vi "09_combined_example.vi"() -> ()   [LabVIEW 2018, in "LV-0mq-Julia_roundtrip-lib.lvlib" / "LV2Julia_examples.lvlib"]
uses:
  LV2Julia_examples.lvlib
  LV2Julia_core/VIs/Server or client state.ctl
  LV2Julia_core/VIs/detailed error info.ctl
  LV2Julia_core/VIs/StackFrame.ctl
  simple examples functions.ctl
  LV2Julia_core/VIs/Commands.ctl
  edf81fa3-46bf-427f-9605-85b461656974.vi
  29886417-d43f-41fb-9c0c-469db3f8c96d.vi
  3fe35f36-217a-40a5-a789-8326c52a1f5c.vi
  35a44a82-786b-41ea-be73-9a4468e4df9d.vi
  edf81fa3-46bf-427f-9605-85b461656974.vi/d78438c1-e9c2-4049-8a01-ea359766d27e.vi
  29886417-d43f-41fb-9c0c-469db3f8c96d.vi/726a0e03-44e9-4b5b-8c33-3fdb3adf96f2.vi
  3fe35f36-217a-40a5-a789-8326c52a1f5c.vi/be66880e-2f9f-43fa-8a25-3020ddce25df.vi
  35a44a82-786b-41ea-be73-9a4468e4df9d.vi/e765cad0-9840-4168-a112-da73896eb643.vi
  35a44a82-786b-41ea-be73-9a4468e4df9d.vi/f3238023-a8b3-435f-be8b-4be774610aa1.vi
  edf81fa3-46bf-427f-9605-85b461656974.vi/d78438c1-e9c2-4049-8a01-ea359766d27e.vi/edf13171-bb8c-4b0e-8a13-cfaee6010a46.vi
  29886417-d43f-41fb-9c0c-469db3f8c96d.vi/726a0e03-44e9-4b5b-8c33-3fdb3adf96f2.vi/e7bf7d0e-5fa3-492d-91d8-494ec4c78bd1.vi
  29886417-d43f-41fb-9c0c-469db3f8c96d.vi/726a0e03-44e9-4b5b-8c33-3fdb3adf96f2.vi/bcfacdb4-d734-4844-97c1-59f988d0ab4b.vi
  29886417-d43f-41fb-9c0c-469db3f8c96d.vi/726a0e03-44e9-4b5b-8c33-3fdb3adf96f2.vi/27f03db2-f0c9-44fc-95a3-84f8622bf8b3.vi
  3fe35f36-217a-40a5-a789-8326c52a1f5c.vi/be66880e-2f9f-43fa-8a25-3020ddce25df.vi/b22e8afe-8408-4b96-ba33-df0573f8bda9.vi
  3fe35f36-217a-40a5-a789-8326c52a1f5c.vi/be66880e-2f9f-43fa-8a25-3020ddce25df.vi/973810d6-8273-42e9-becd-a912c4fb1f62.vi
  3fe35f36-217a-40a5-a789-8326c52a1f5c.vi/be66880e-2f9f-43fa-8a25-3020ddce25df.vi/742d8af4-4bb6-4e08-85d7-281a839dc2ce.vi
  35a44a82-786b-41ea-be73-9a4468e4df9d.vi/e765cad0-9840-4168-a112-da73896eb643.vi/dc34fd2d-f794-448f-aba6-043ae9d4d40f.vi
  35a44a82-786b-41ea-be73-9a4468e4df9d.vi/e765cad0-9840-4168-a112-da73896eb643.vi/fa03b5a1-01ca-4e07-872a-a6bd434a2e33.vi
  edf81fa3-46bf-427f-9605-85b461656974.vi/d78438c1-e9c2-4049-8a01-ea359766d27e.vi/edf13171-bb8c-4b0e-8a13-cfaee6010a46.vi/3952a552-d88b-4b70-b2de-8936c03ae8d7.vi
  35a44a82-786b-41ea-be73-9a4468e4df9d.vi/e765cad0-9840-4168-a112-da73896eb643.vi/dc34fd2d-f794-448f-aba6-043ae9d4d40f.vi/6b1990a7-d1b9-4824-acae-e43fafbf4c5e.vi
  LV2Julia_core/VIs/jl-scripts path.vi
  LV2Julia_core/VIs/check ID validity.vi
  LV2Julia_core/VIs/bindata_descr to JSON.vi
  LV2Julia_core/VIs/check cluster field names.vi
  LV2Julia_core/VIs/concat JSON.vi
  LV2Julia_core/VIs/build request.vi
  LV2Julia_core/VIs/Parse server response.vi
  LV2Julia_core/VIs/log jl exceptions.vi
  <vilib>/Utility/error.llb/Error Cluster From Error Code.vi
  LV2Julia_core/LV2Julia_core.lvlib
  <vilib>/measure/NI_MABase.lvlib
panel:
  out "ZMQ timeout":bool
  out "Julia script file path":path
  out "temporary script path":path
  out "Jl Server state":T1
  in  "execution control pages":enum32{"Start", "go - test"}(tab)
  in  "go":bool caption="go (Julia Server started externally)"
  in  "Start with Julia":bool caption="Start Julia Server and go"
  in  "ZMQ endpoint":string="tcp://127.0.0.1:5555"
  in  "p":dbl=1.0
  in  "fn":T2 caption="select function at Server" items=["arr_amplitude", "arr_length", "arr_mean", "arr_median", "arr_rms", "vec_amplify", "vec_attenuate", "vec_power"]
  in  "trim @ begin":dbl
  in  "trim @ end":dbl
  in  "Group":T3(tab)
  out "Server response":dbl
  out "data received plot":dbl[](graph)
  out "data received":dbl[](array[numeric]) format="%.3f"
  out "RMS":dbl
  out "detailed error info":T4
  out "current error":errorcluster
  out "final error":errorcluster
  out "short err code":u8
  in  "tones":T6(array[cluster])=[{"frequency"=10.0, "amplitude"=1.0, "phase"=0.0}, {"frequency"=20.0, "amplitude"=0.1, "phase"=0.0}] {"phase" format="%.2p"; "amplitude" format="%0.2p"; "frequency" format="%0.2p"}
  in  "noise (rms)":dbl=0.1 format="%.2p"
  in  "offset":dbl format="%.2p"
  in  "sampling info":cluster{"Fs":dbl, "#s":dbl}={"Fs"=1000.0, "#s"=1000.0} {"Fs" format="%.2p"}
  in  "next":bool
  out "data sent to server":dbl[](graph)
  out "data sent":dbl[](array[numeric]) format="%.3f"
  out "function name":string
  in  "stop this VI only":bool
  in  "stop both this VI and Julia Server":bool
  # "tcp://127.0.0.1:5555 \nfor local Julia Server\n\nFor a Julia Server running on a separate computer,  you probably must use an IPv4 address in numeric form (not a DNS name) - see https://stackoverflow.com/questions/6024003/why-doesnt-zeromq-work-on-localhost.\n\nThis control only used if Julia Server is not being started by this VI."
  # "generate sample array"
  # "function and parameter"
  # "enter a negative or a large positive value to cause an exception"
  # "data returned by server"
  # "data sent to server"
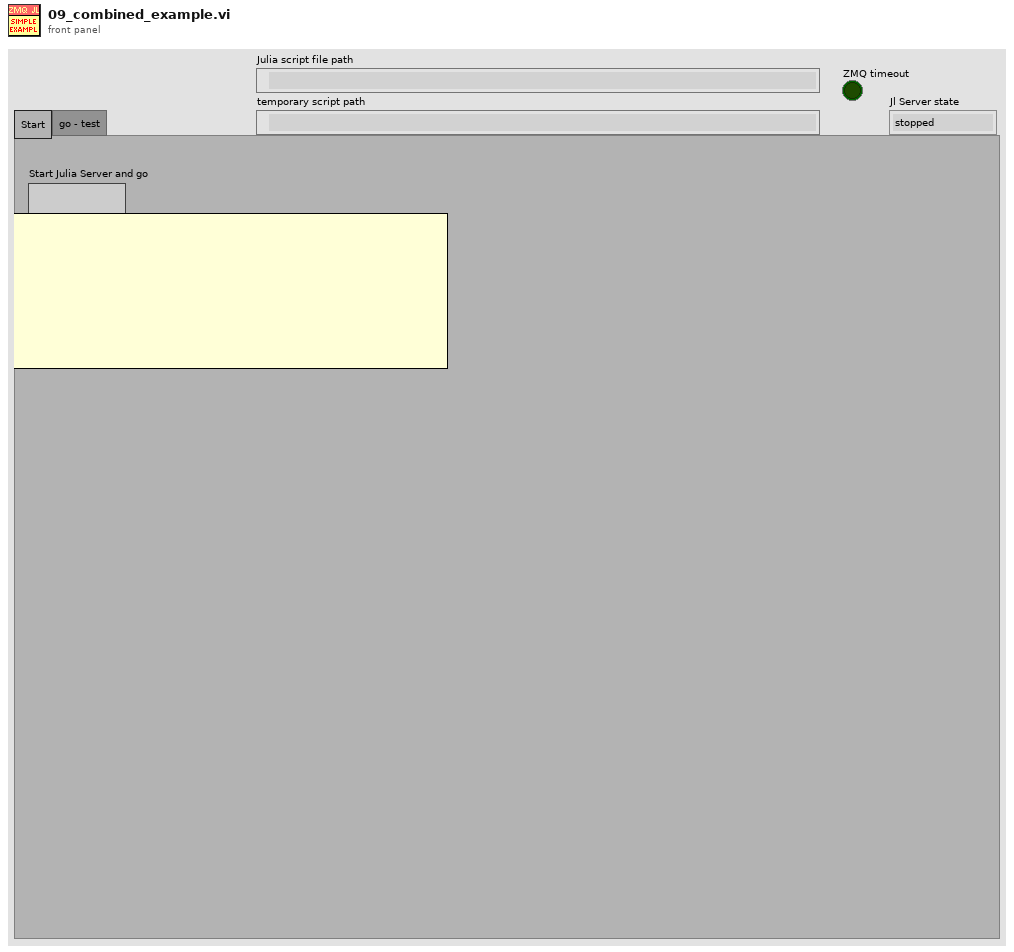
[diagram p1: front panel]
types:
  T1 = typedef "LV-0mq-Julia_roundtrip-lib.lvlib/LV2Julia_core.lvlib/Server or client state.ctl" = enum16{"stopped", "running", "unknown"}
  T2 = typedef "LV-0mq-Julia_roundtrip-lib.lvlib/LV2Julia_examples.lvlib/simple examples functions.ctl" = u16
  T3 = enum32{"fns returning scalar", "fns returning vector", "error"}
  T4 = typedef "LV-0mq-Julia_roundtrip-lib.lvlib/LV2Julia_core.lvlib/detailed error info.ctl" = cluster{"exception_or_info":string, "trace":T5[]}
  T5 = typedef "LV-0mq-Julia_roundtrip-lib.lvlib/LV2Julia_core.lvlib/StackFrame.ctl" = cluster{"frame_summary":string, "func":string, "linfo":string, "file":string, "line":i32, "pointer":u64, "from_c":bool, "inlined":bool}
  T6 = cluster{"frequency":dbl, "amplitude":dbl, "phase":dbl}[]
  T7 = typedef "LV-0mq-Julia_roundtrip-lib.lvlib/LV2Julia_core.lvlib/Commands.ctl" = enum16{"Start Jl-server & Init LV-client", "Send request & Get response ", "Stop Jl-server & Cleanup LV-client", "Cleanup LV-client", "Start Jl-server", "Stop Jl-server", "Init LV-Client", "Cleanup LV-Client", "(not allowed)", "Set LV Client state", "Set Jl Server state", "set ZMQ timeout", "read ZMQ timeout", "read-out state"}
  T8 = enum8{"Enabled", "Disabled", "Disabled and Grayed Out"}
  T9 = typedef "LV-0mq-Julia_roundtrip-lib.lvlib/LV2Julia_core.lvlib/Bindata&description.ctl" = cluster{"bindata_descr":T10[], "bindata":u8[]}
  T10 = typedef "LV-0mq-Julia_roundtrip-lib.lvlib/LV2Julia_core.lvlib/Bindata description.ctl" = cluster{"nofbytes":i32, "numtype":string, "start":i32, "arrdims":i32[], "kwarg_name":string, "category":string}
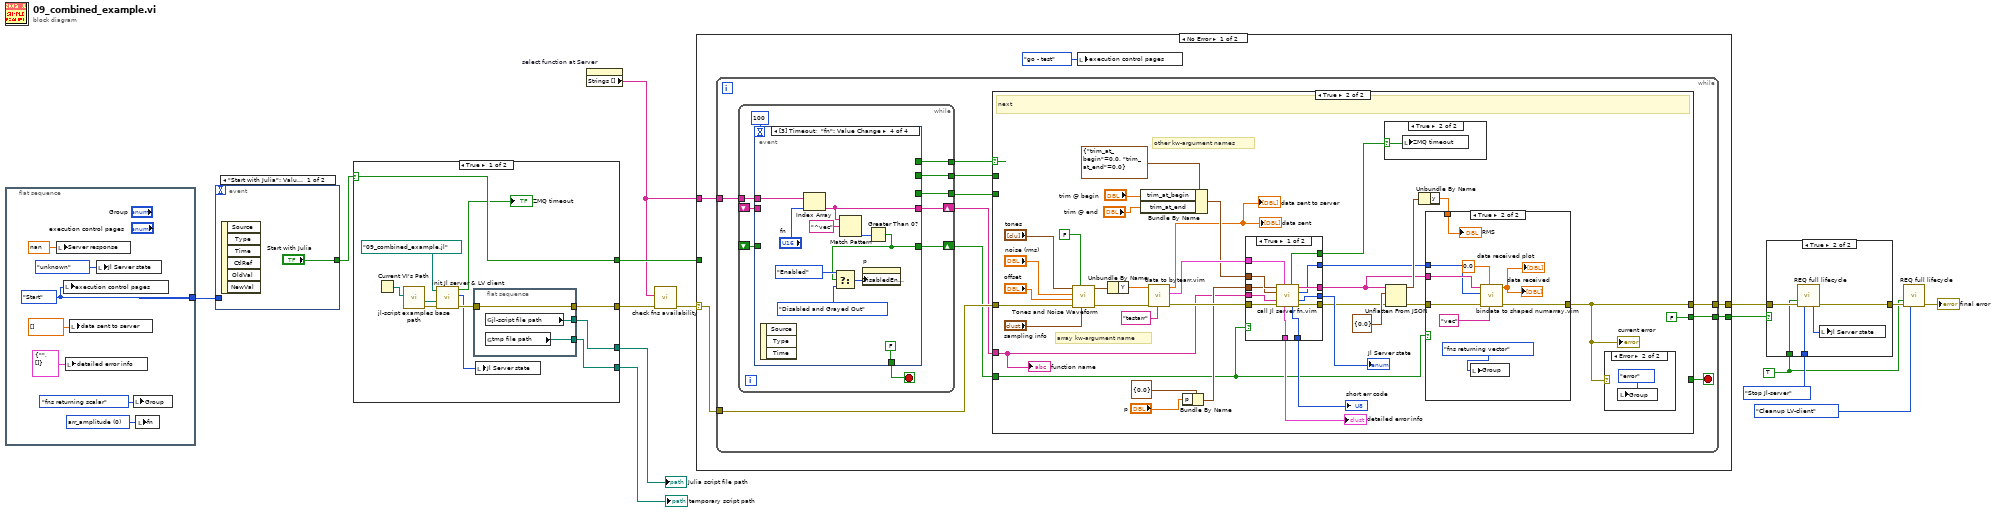
[diagram p0: block diagram]
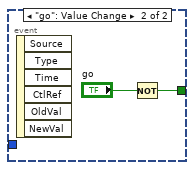
[diagram p2: hidden frame]
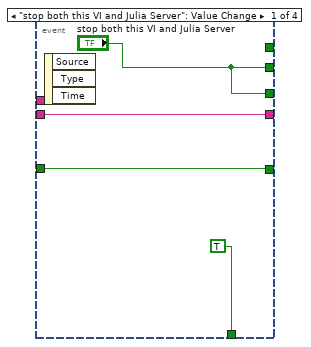
[diagram p3: hidden frame]
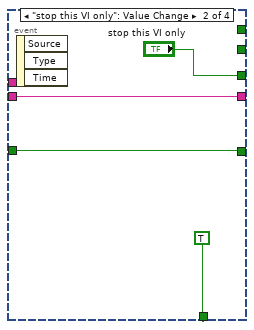
[diagram p4: hidden frame]
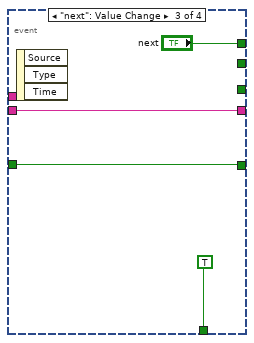
[diagram p5: hidden frame]
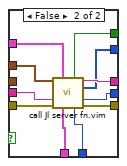
[diagram p7: hidden frame]
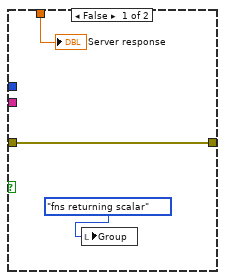
[diagram p9: hidden frame]
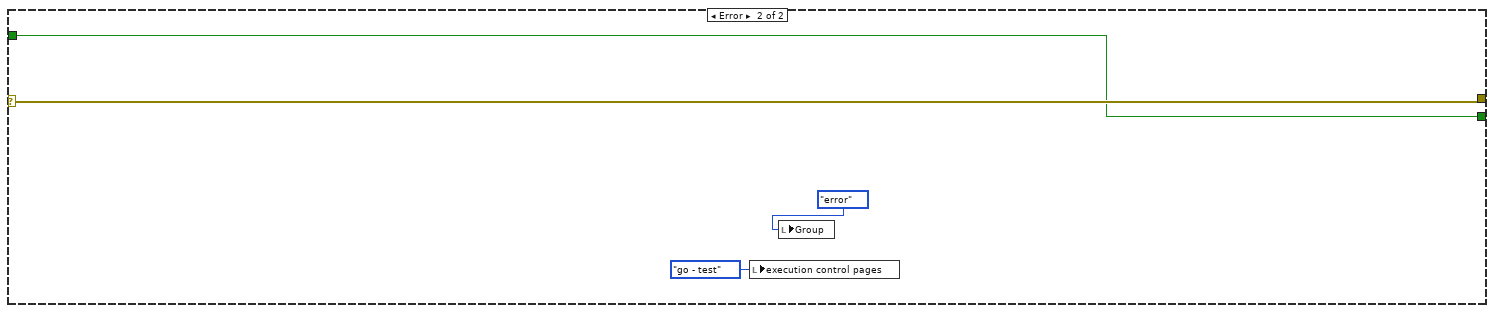
[diagram p11: hidden frame]
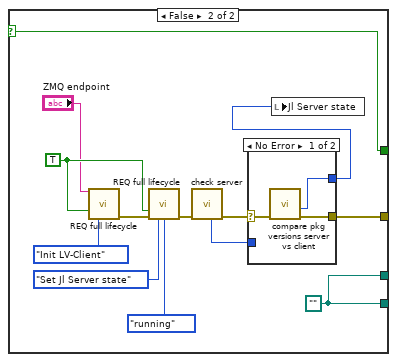
[diagram p12: hidden frame]
diagram:
  w10 = TRUE ("Force command")
  n1 = flat-sequence {
    tunnel: [w22] -> w6
    frame #0 {
      w16 = T2 0 items=["arr_amplitude", "arr_length", "arr_mean", "arr_median", "arr_rms", "vec_amplify", "vec_attenuate", "vec_power"] ("fn")
      w22 = enum32{"Start", "go - test", "finish"}."Start" ("execution control pages")
      n2 = local write "Server response"(nan ("Server response")) -> ()
      n3 = local write "execution control pages"(w22) -> ()
      n4 = local write "detailed error info"(T4 {"exception_or_info"="", "trace"=[]} ("detailed error info")) -> ()
      n5 = local write "data sent to server"(dbl[] []) -> ()
      n6 = local write "Jl Server state"(Server_or_client_state."unknown" ("Jl Server state out")) -> ()
      n7 = local write "Group"(T3."fns returning scalar" ("Group")) -> ()
      n8 = local write "fn"(w16) -> ()
    }
  }
  n9 = event shown="[0] \"Start with Julia\": Value Change" {
    selector: _ -> [_ _]
    dyn-events: _ -> [_ _]
    timeout: _ -> [_ _]
    tunnel: ["Start with Julia" w24] -> w8
    tunnel: w6 -> [_ _]
    event "Start with Julia": Value Change {
      n10 = event-data() -> ()  [unwired: 1 in, 6 out]
    }
    event "go": Value Change {
      n11 = event-data() -> ()  [unwired: 1 in, 6 out]
      n12 = Not(x="go") -> (.not. x?=w24:bool)
    }
  }
  n13 = case shown="True" w8 {
    selector: w8 -> [w36 w48]
    tunnel: [w35 w42] -> w5
    tunnel: [w36 w48] -> w7
    tunnel: [w34 w45] -> w1
    tunnel: [w33 w45] -> w2
    frame True {
      n14 = Current VI's Path() -> (path=w28:path)
      n15 = call "jl-script examples base path.vi"("calling example VI path"=w28) -> ("error out"=w27:errorcluster, "jl-script-examples base path"=w26:path)  [unwired: 9 in]
      n16 = call "init Jl server & LV client.vi"("error in (no error)"=w27, "Base path (not a path)"=w26, "Julia user functions script"=path "09_combined_example.jl") -> ("error out"=w30:errorcluster, "Jl Server state out"=w29:T1, "timeout?"=→"ZMQ timeout":bool)  [unwired: 6 in]
      n17 = flat-sequence {
        tunnel: [w39] -> w35
        tunnel: w30 -> [w39]
        tunnel: [w38] -> w34
        tunnel: [w37] -> w33
        frame #0 {
          n18 = global read "jl-scripts path.vi" "jl-script file path"() -> (w38:path)
          n19 = global read "jl-scripts path.vi" "tmp file path"() -> (w37:path)
        }
      }
      n20 = local write "Jl Server state"(w29) -> ()
    }
    frame False {
      w45 = path ""
      w50 = TRUE ("Force command")
      n21 = call "REQ full lifecycle.vi"("ZMQ endpoint"="ZMQ endpoint", "Force command"=w50, "command"=Commands."Init LV-Client") -> ("error out"=w47:errorcluster)  [unwired: 6 in, 6 out]
      n22 = call "REQ full lifecycle.vi"("Force command"=w50, "error in"=w47, "command"=Commands."Set Jl Server state", "Jl Server state in"=Server_or_client_state."running") -> ("error out"=w46:errorcluster)  [unwired: 5 in, 6 out]
      n23 = call "check server.vi"("error in"=w46) -> ("error out"=w43:errorcluster, "Jl Server state out"=w41:T1)  [unwired: 6 in, 3 out]
      n24 = case shown="No Error" w43 {
        selector: w43 -> [w55 w57]
        tunnel: [w54 w57] -> w42
        tunnel: [w53 w56] -> w40
        tunnel: w41 -> [_ w56]
        frame No Error {
          n25 = call "compare pkg versions server vs client.vi"("error in (no error)"=w55) -> ("error out"=w54:errorcluster, "Jl Server state out"=w53:T1)  [unwired: 4 in, 5 out]
        }
        frame Error {
        }
      }
      n26 = local write "Jl Server state"(w40) -> ()
    }
  }
  "temporary script path" <- w2
  "Julia script file path" <- w1
  n27 = property on="select function at Server" class="Ring (strict)"() -> ("Strings []"=w3:string[])  [unwired: 2 in, 2 out]
  n28 = call "check fns availability.vi"("error in (no error)"=w5, "fns list is"=w3) -> ("error out"=w4:errorcluster)  [unwired: 3 in, 6 out]
  n29 = case shown="No Error" w4 {
    selector: w4 -> [w61 w183]
    tunnel: [w62 w183] -> w15
    tunnel: [w60 w182] -> w9
    tunnel: w3 -> [w59 _]
    tunnel: w7 -> [_ w182]
    frame No Error {
      n30 = while {
        tunnel: w61 -> [w71]
        tunnel: [w72] -> w62
        tunnel: [w68] -> w60
        tunnel: w59 -> [w66]
        stop <- w69 stop-if-true
        n31 = while {
          tunnel: [w82] -> w70
          tunnel: [w81] -> w67
          tunnel: w66 -> [w78]
          shift-right: [w77] -> w65
          shift-left: _ -> [w74]
          shift-right: [w76] -> w64
          shift-left: _ -> [w75]
          tunnel: [w73] -> w63
          stop <- w80 stop-if-true
          n32 = event shown="[3] Timeout;  \"fn\": Value Change" {
            selector: _ -> [_ _ _ _]
            dyn-events: _ -> [_ _ _ _]
            timeout: 100 -> [_ _ _ _]
            tunnel: ["stop both this VI and Julia Server" _ _ _] -> w81
            tunnel: [_ _ "next" _] -> w82
            tunnel: [TRUE TRUE TRUE FALSE] -> w80
            tunnel: w78 -> [_ _ _ w98]
            tunnel: [w84 w88 w92 w97] -> w77
            tunnel: [w85 w89 w91 w96] -> w76
            tunnel: w75 -> [w85 w89 w91 _]
            tunnel: w74 -> [w84 w88 w92 _]
            tunnel: ["stop both this VI and Julia Server" "stop this VI only" _ _] -> w73
            event "stop both this VI and Julia Server": Value Change {
              n33 = event-data() -> ()  [unwired: 1 in, 3 out]
            }
            event "stop this VI only": Value Change {
              n34 = event-data() -> ()  [unwired: 1 in, 3 out]
            }
            event "next": Value Change {
              n35 = event-data() -> ()  [unwired: 1 in, 3 out]
            }
            event Timeout; Value Change {
              n36 = event-data() -> ()  [unwired: 1 in, 3 out]
              n37 = Index Array(array=w98, index="fn") -> (element=w96:string)
              n38 = Match Pattern(string=w96, regular expression="^vec") -> (offset past match=w102:i32)  [unwired: 1 in, 3 out]
              n39 = Greater Than 0?(x=w102) -> (x > 0?=w97:bool)
              n40 = Select(t=T8."Enabled" ("Disabled"), s=w97, f=T8."Disabled and Grayed Out" ("Disabled")) -> (s? t:f=w104:T8)
              n41 = property on="p" class="DigNum (strict)"("DisabledEnum"=w104) -> ()  [unwired: 2 in, 2 out]
            }
          }
        }
        n42 = case shown="True" w70 {
          tunnel: [w107 w123] -> w72
          tunnel: w71 -> [w107 w128]
          tunnel: [w106 w127] -> w69
          tunnel: w63 -> [w106 _]
          tunnel: [w105 w127] -> w68
          tunnel: w67 -> [w105 _]
          tunnel: w65 -> [_ w109]
          tunnel: w64 -> [_ w111]
          frame False {
            # "stop"
          }
          frame True {
            w127 = FALSE ("stop this VI only")
            # "other kw-argument names"
            # "array kw-argument name"
            # "next"
            n43 = call <vilib>:"Tones and Noise Waveform.vi"("sampling info"="sampling info", "reset signal"=FALSE, "error in (no error)"=w128, "offset"="offset", "noise (rms)"="noise (rms)", "tones"="tones") -> ("error out"=w129:errorcluster, "signal out"=w135:waveform(dbl))  [unwired: 4 in]
            n44 = Unbundle By Name(w135) -> ("Y"=w130:dbl[])
            n45 = Bundle By Name(cluster=cluster{"trim_at_begin":dbl, "trim_at_end":dbl} {"trim_at_begin"=0.0, "trim_at_end"=0.0}, "trim_at_begin"="trim @ begin", "trim_at_end"="trim @ end") -> (w113:cluster{"trim_at_begin":dbl, "trim_at_end":dbl})
            n46 = call "data to bytearr.vim"("kwarg_name"="testarr", "error in (no error)"=w129, "data in"=w130) -> ("error out"=w121:errorcluster, "Bindata & descr out"=w114:T9, "flattened data out"=→"data sent" →"data sent to server":dbl[])  [unwired: 6 in]
            n47 = Bundle By Name(cluster=cluster{"p":dbl} {"p"=0.0}, "p"="p") -> (w112:cluster{"p":dbl})
            n48 = case shown="True" w109 {
              tunnel: w121 -> [w154 w165]
              tunnel: [w153 w164] -> w120
              tunnel: [w152 w163] -> w119
              tunnel: [w151 w162] -> w118
              tunnel: [w150 w161] -> w117
              tunnel: [w149 w160] -> w116
              tunnel: [w148 w159] -> w115
              tunnel: w114 -> [w147 w158]
              tunnel: w113 -> [w146 w157]
              tunnel: w112 -> [w145 _]
              tunnel: w111 -> [w144 w156]
              tunnel: [w143 w155] -> w110
              frame True {
                n49 = call "call Jl server fn.vim"("Arguments 1"=w146, "Bindata & descr in"=w147, "Arguments 2"=w145, "fun2call"=w144, "error in (no error)"=w154) -> ("timeout?"=w148:bool, "JSON received"=w150:string, "binary data received"=w149:u8[], "Jl Server state out"=w152:T1, "detailed error info"=w153:T4, "return code"=w143:u8, "error out"=w151:errorcluster)  [unwired: 4 in]
              }
              frame False {
                n50 = call "call Jl server fn.vim"("Arguments 1"=w157, "Bindata & descr in"=w158, "fun2call"=w156, "error in (no error)"=w165) -> ("timeout?"=w159:bool, "JSON received"=w161:string, "binary data received"=w160:u8[], "Jl Server state out"=w163:T1, "detailed error info"=w164:T4, "return code"=w155:u8, "error out"=w162:errorcluster)  [unwired: 5 in]
              }
            }
            "short err code" <- w110
            "Jl Server state" <- w119
            "detailed error info" <- w120
            n51 = case shown="True" w115 {
              selector: w115 -> [_ w166]
              frame False {
              }
              frame True {
                n52 = local write "ZMQ timeout"(w166) -> ()
              }
            }
            n53 = Unflatten From JSON(JSON string=w117, type and defaults=cluster{"y":dbl} {"y"=0.0} ("parsed response"), error in (no error)=w118) -> (value=w141:cluster{"y":dbl}, error out=w124:errorcluster)  [unwired: 4 in]
            n54 = Unbundle By Name(w141) -> ("y"=w122:dbl)
            n55 = case shown="True" w109 {
              tunnel: w124 -> [w169 w177]
              tunnel: [w169 w176] -> w123
              tunnel: w116 -> [_ w170]
              tunnel: w117 -> [_ w171]
              tunnel: w122 -> [w167 w173]
              frame False {
                n56 = local write "Group"(T3."fns returning scalar" ("Group")) -> ()
                "Server response" <- w167
              }
              frame True {
                n57 = local write "Group"(T3."fns returning vector" ("Group")) -> ()
                n58 = call "bindata to shaped numarray.vim"("name"="vec" ("kwarg_name"), "element type"=0.0 ("data type"), "error in (no error)"=w177, "binary data"=w170, "JSON in"=w171) -> ("error out"=w176:errorcluster, "numarray 1D"=→"data received plot" →"data received":dbl[])  [unwired: 3 in, 2 out]
                "RMS" <- w173
              }
            }
            "current error" <- w123
            n59 = case shown="Error" w123 {
              frame No Error {
              }
              frame Error {
                n60 = local write "Group"(T3."error" ("Group")) -> ()
              }
            }
            "function name" <- w111
          }
        }
      }
      n61 = local write "execution control pages"(enum32{"Start", "go - test", "finish"}."go - test" ("execution control pages")) -> ()
    }
    frame Error {
      n62 = local write "execution control pages"(enum32{"Start", "go - test", "finish"}."go - test" ("execution control pages")) -> ()
      n63 = local write "Group"(T3."error" ("Group")) -> ()
    }
  }
  n64 = case shown="True" w9 {
    tunnel: w15 -> [w184 w189]
    tunnel: Commands."Stop Jl-server" ("command") -> [_ w188]
    tunnel: [w184 w187] -> w13
    tunnel: w10 -> [_ w186]
    frame False {
    }
    frame True {
      n65 = call "REQ full lifecycle.vi"("Force command"=w186, "error in"=w189, "command"=w188) -> ("Jl Server state out"=w185:T1, "error out"=w187:errorcluster)  [unwired: 6 in, 5 out]
      n66 = local write "Jl Server state"(w185) -> ()
    }
  }
  n67 = call "REQ full lifecycle.vi"("Force command"=w10, "error in"=w13, "command"=Commands."Cleanup LV-client") -> ("error out"=→"final error":errorcluster)  [unwired: 6 in, 6 out]
